vi "brokenTask.vi"(8 "error in (no error)":errorcluster, 10 "ITaskChannel":refnum<class "ITaskChannel.lvclass">, 11 "ITask in":refnum<class "ITask.lvclass">) -> (0 "error out":errorcluster, 3 "ITask out":refnum<class "ITask.lvclass">)   [LabVIEW 2023, in "TaskMock.lvclass"]
uses:
  TaskMock.lvclass
  TaskMock.lvclass/TaskMock.ctl
  source/BoolNotifierTaskChannel/BoolNotifierTaskChannel.lvclass
  source/ITask/ITask.lvclass
  source/ITaskChannel/ITaskChannel.lvclass
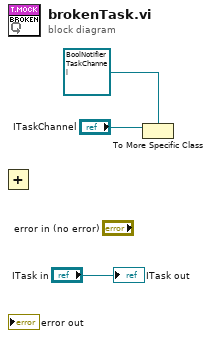
[diagram p0: block diagram]
diagram:
  n1 = Add() -> ()  [unwired: 2 in, 1 out]
  n2 = To More Specific Class(target class=refnum<class "BoolNotifierTaskChannel.lvclass"> refnum ("TLC_Daemon.lvlib:BoolNotifierTaskChannel.lvclass"), reference="ITaskChannel") -> ()  [unwired: 1 in, 2 out]
  "ITask out" <- "ITask in"
